vi "configure.vi"(8 "error in (no error)":errorcluster, 9 "Value":i32, 10 "ILC":refnum<class "ILC.lvclass">, 11 "ConfigureILCDIStrategy in":refnum<class "ConfigureILCDIStrategy.lvclass">) -> (0 "error out":errorcluster, 3 "ConfigureILCDIStrategy out":refnum<class "ConfigureILCDIStrategy.lvclass">)   [LabVIEW 2015, in "ConfigureILCDIStrategy.lvclass"]
uses:
  ConfigureILCDIStrategy/ConfigureILCDIStrategy.lvclass
  <userlib>/Common/ILC/ILC/ILC.lvclass
  ConfigureILCDIStrategy/ConfigureILCDIStrategy.lvclass/ConfigureILCDIStrategy.ctl
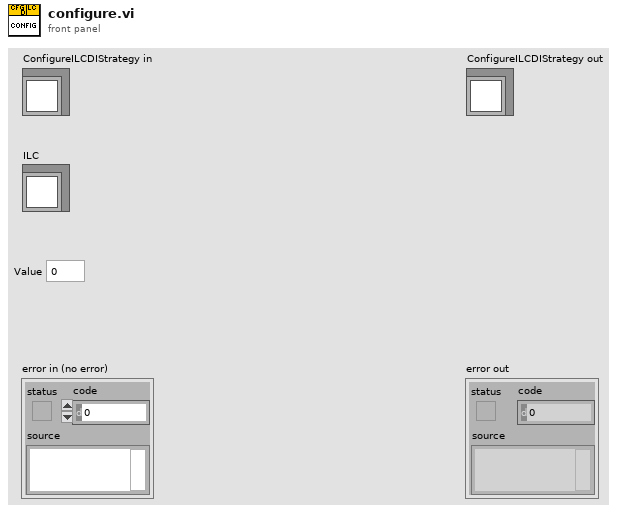
[diagram p1: front panel]
types:
  T1 = typedef "ILCBTTypedefs.lvlib/Digital Signal Level.ctl" = enum16{"Low", "High"}
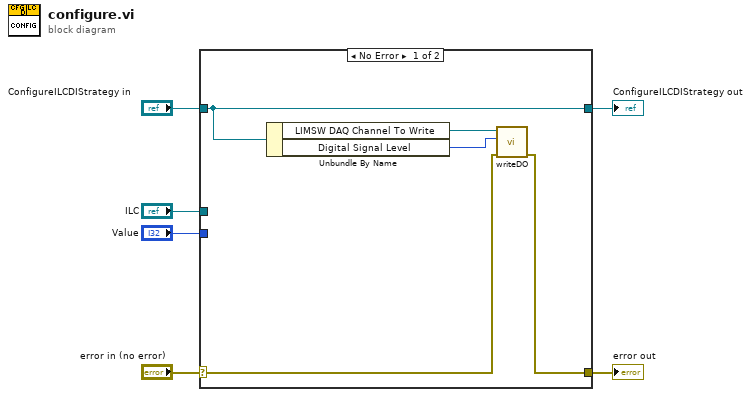
[diagram p0: block diagram]
diagram:
  n1 = case shown="No Error" "error in (no error)" {
    selector: "error in (no error)" -> [w8 w13]
    tunnel: [w7 w13] -> w5
    tunnel: [w10 w12] -> w3
    tunnel: "ConfigureILCDIStrategy in" -> [w10 w12]
    tunnel: "ILC" -> [_ _]
    tunnel: "Value" -> [_ _]
    frame No Error {
      n2 = Unbundle By Name(w10) -> ("LIMSW DAQ Channel To Write"=w9:refnum<k21>, "Digital Signal Level"=w11:T1)
      n3 = call "writeDO.vi"("error in"=w8, "Digital Signal Level"=w11, "DAQmx Global Channel"=w9) -> ("error out"=w7:errorcluster)  [unwired: 8 in]
    }
    frame Error {
    }
  }
  "error out" <- w5
  "ConfigureILCDIStrategy out" <- w3
